vi "Init ADC.vi"(8 "error in (no error)":errorcluster, 11 "ADS1115 in":refnum<class "Grove An In ADS1115.lvclass">) -> (0 "error out":errorcluster, 3 "ADS1115 out":refnum<class "Grove An In ADS1115.lvclass">)   [LabVIEW 2020, in "CTI-Peripheral.lvlib" / "Grove An In ADS1115.lvclass"]
uses:
  Grove An In ADS1115.lvclass
  Grove An In ADS1115.lvclass/Grove An In ADS1115.ctl
  CTI/I2C Connection/I2C Connection.lvclass/I2C Connection.ctl
  CTI/Session/I2C Write Data.vi
  CTI/I2C Connection/I2C Connection.lvclass
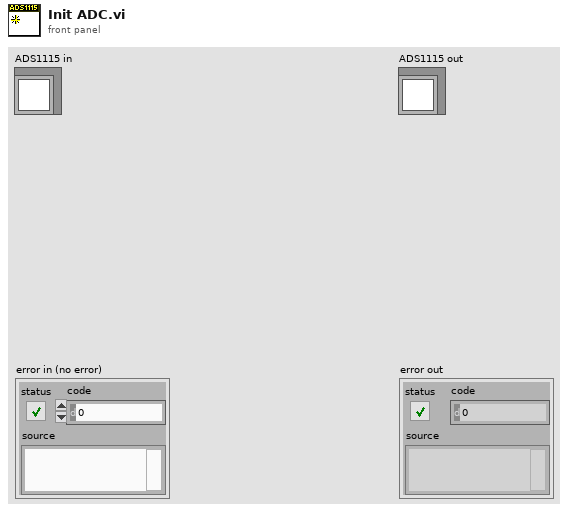
[diagram p1: front panel]
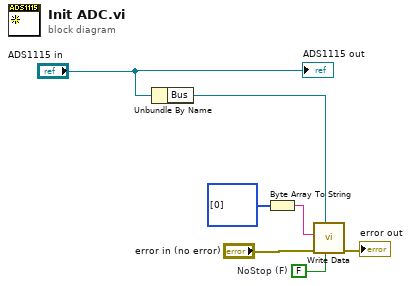
[diagram p0: block diagram]
diagram:
  w4 = FALSE  # NoStop (F)
  n1 = Unbundle By Name("ADS1115 in") -> ("Bus"=w6:refnum<class "I2C Connection.lvclass">)
  n2 = Byte Array To String(unsigned byte array=u8[] [0]) -> (string=w3:string)
  n3 = call "Write Data.vi"("NoStop (F)"=w4, "I2C Connection"=w6, "error in (no error)"="error in (no error)", "Data"=w3) -> ("error out"=→"error out":errorcluster)  [unwired: 7 in]
  "ADS1115 out" <- "ADS1115 in"
